vi "Find VI with Focus - Test Support - Teardown.vi"(8 "error in (no error)":errorcluster, 11 "VI Renum":refnum<vi>) -> (0 "error out":errorcluster)   [LabVIEW 2009]
doc: "This VI closes the Test Support's front panel and reference."
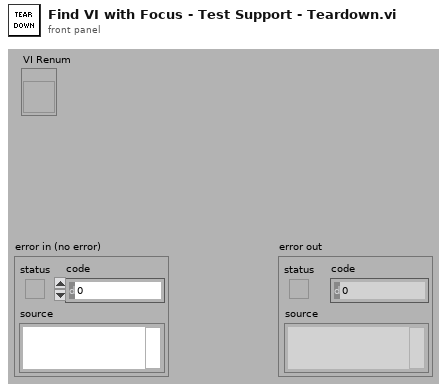
[diagram p1: front panel]
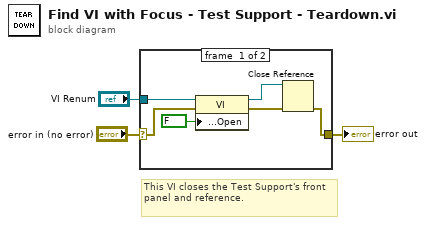
[diagram p0: block diagram]
diagram:
  # "This VI closes the Test Support's front panel and reference."
  n1 = case shown="No Error" "error in (no error)" {
    selector: "error in (no error)" -> [w4 w10]
    tunnel: "VI Renum" -> [w9 _]
    tunnel: [w5 w10] -> w1
    frame #0 {
      n2 = property class="VI"(reference=w9, error in=w4, "Front Panel.Open"=FALSE ("Front Panel Window:Open")) -> (reference out=w7:refnum<vi>, error out=w6:errorcluster)
      n3 = Close Reference(reference=w7, error in (no error)=w6) -> (error out=w5:errorcluster)
    }
    frame #1 {
    }
  }
  "error out" <- w1
